vi "Goal Align.vi"(6 "last":bool) -> (1 "Right":dbl, 2 "Left":dbl)   [LabVIEW 2015]
uses:
  Robot Global Data.vi
  <vilib>/addons/control/pid/pid.llb/PID (DBL).vi
  <vilib>/addons/control/pid/NI_PID_pid.lvlib
  navX/navX Library v2/navX Library v2.lvlib
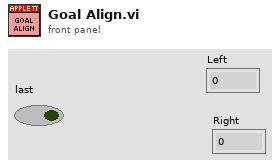
[diagram p1: front panel]
types:
  T1 = typedef "navX Library v2.lvlib/Z900_navX_DeviceTypeDef.ctl" = cluster{"Interface":cluster{"Protocol":T2, "Update Rate (4Hz-60Hz)":u8, "navX Open TypeDef":variant}, "Notify Packet":refnum<notifier>, "Loop VI Refnum":refnum<vi>, "Ready to Close Occurrence Refnum":refnum<k4>}
  T2 = typedef "navX Library v2.lvlib/Z900_navX_ProtocolTypeDef.ctl" = enum16{"SERIAL", "I2C", "SPI"}
  T3 = cluster{"Yaw":dbl, "Roll":dbl, "Pitch":dbl, "Heading":dbl, "Fused Heading":dbl}
  T4 = cluster{"proportional gain (Kc)":dbl, "integral time (Ti, min)":dbl, "derivative time (Td, min)":dbl}
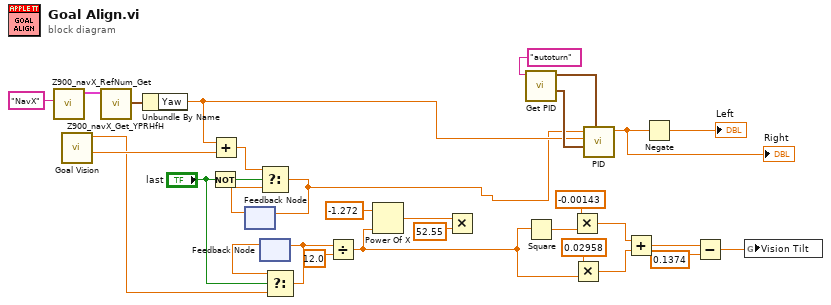
[diagram p0: block diagram]
diagram:
  n1 = call "Z900_navX_RefNum_Get.vi"("refnum name"="NavX") -> ("navX Device"=w26:T1)  [unwired: 9 in, 1 out]
  n2 = call "Goal Vision.vi"() -> ("X Angle"=w22:dbl, "Distance (in)"=w14:dbl)  [unwired: 8 in, 1 out]
  n3 = call "Z900_navX_Get_YPRHfH.vi"("navX Device"=w26) -> ("YRPHfH"=w24:T3)  [unwired: 7 in, 3 out]
  n4 = Unbundle By Name(w24) -> ("Yaw"=w21:dbl)
  n5 = Not(x="last") -> (.not. x?=w28:bool)
  n6 = Add(x=w21, y=w22) -> (x+y=w23:dbl)
  n7 = feedback #1() -> (w27:dbl)  [unwired: 1 in]
  n8 = Select(t=w23, s=w28, f=w27) -> (s? t:f=w1:dbl)
  n9 = feedback-in #1(w1) -> ()
  n10 = feedback #2() -> (w19:dbl)  [unwired: 1 in]
  n11 = Select(t=w19, s="last", f=w14) -> (s? t:f=w16:dbl)
  n12 = feedback-in #2(w16) -> ()
  n13 = Divide(x=w16, y=12.0) -> (x/y=w5:dbl)
  n14 = Power Of X(1:w5, 2:-1.272 ("y")) -> (0:w3:dbl)
  n15 = Multiply(x=w3, y=52.55) -> ()  [unwired: 1 out]
  n16 = call "Get PID.vi"("Subsystem"="autoturn") -> ("PID Gains"=w31:T4, "output range"=w30:cluster{"output high":dbl, "output low":dbl})  [unwired: 8 in]
  n17 = Square(x=w5) -> (x^2=w13:dbl)
  n18 = Multiply(x=-0.00143, y=w13) -> (x*y=w10:dbl)
  n19 = Multiply(x=0.02958, y=w5) -> (x*y=w9:dbl)
  n20 = call-poly <vilib>:"PID.vi"("output range"=w30, "PID gains"=w31, "process variable"=w21, "setpoint"=w1) -> ("output"=w17:dbl)  [unwired: 6 in, 1 out]
  "Right" <- w17
  n21 = Add(x=w10, y=w9) -> (x+y=w8:dbl)
  n22 = Negate(x=w17) -> (-x=→"Left":dbl)
  n23 = Subtract(x=w8, y=0.1374) -> (x-y=w6:dbl)
  n24 = global write "Robot Global Data.vi" "Vision Tilt"(w6) -> ()
